vi "Raman Live Tool Set v10.2.2.vi"(1 "Exit":bool, 2 "LiveData":dbl[][](array[numeric]), 3 "RemoteIndicator":bool) -> ()   [LabVIEW 2010]
uses:
  subvi/_TypeDefs/MapFunctions.ctl
  <vilib>/Utility/miscctls.llb/LVPointTypeDef.ctl
  <vilib>/Utility/miscctls.llb/LVStringsAndValuesArrayTypeDef.ctl
  <vilib>/Utility/inputDevices.llb/closeKeyboard.vi
  <vilib>/Utility/inputDevices.llb/keyboardAcquire.vi
  <vilib>/Utility/file.llb/Read From Spreadsheet File (string).vi
  <vilib>/Analysis/NI_AALBase.lvlib
panel:
  in  "MapFunction":T1 caption="Mapping function" items=["Total"=0, "Peak"=4, "Area"=2, "Value"=1, "Ratio"=3]
  in  "CreateMap":bool
  in  "SpectrumCoerce":dbl caption="Limit?"
  out "XY Full Interpol.":cluster{dbl, dbl}[](array[cluster])
  out "Axes":T2
  in  "SpectrumNoise":dbl caption="Noise?"
  in  "SpectrumX":u16(ring) caption="X"
  in  "SpectrumY":u16(ring) caption="Y"
  out "Spectrum":cluster{dbl[], dbl[]}(graph) caption="Current Spectrum"
  in  "MapKeyboard":bool
  in  "MapEditColor":bool caption="Edit Color"
  in  "MapFlipColor":bool caption="Flip Color"
  in  "MapInterpolate":bool
  in  "MapSaveData":bool
  out "Map":dbl[][](graph)
  out "LoadingSpectra":bool
  in  "SourceFile":path caption="Mapping File"
  in  "MapCursorDummy":bool
  out "XY Unique":cluster{"X Unique":dbl[], "Y Unique":dbl[]}
  out "XY Full":cluster{dbl, dbl}[](array[cluster])
  out "Intensities (2D)":dbl[][](array[numeric])
  out "Wavelengths (1D)":dbl[](array[numeric])
  out "MapColorTable":u32[](array[numeric])=[0, 196608, 393216, 589824, 786432, 983040, 1179648, 1376256, 1572864, 1769472, 1966080, 2162688, 2359296, 2555904, 2752512, 2949120, 3145728, 3342336, 3538944, 3735552, 3932160, 4128768, 4325376, 4521984, 4718592, 4915200, 5111808, 5308416, 5505024, 5701632, 5898240, 6094848, 6291456, 6488064, 6684672, 6881280, 7077888, 7274496, 7471104, 7667712, 7864320, 8060928, 8257536, 8454144, 8650752, 8847360, 9043968, 9240576, 9437184, 9633792, 9830400, 10027008, 10223616, 10420224, 10616832, 10813440, 11010048, 11206656, 11403264, 11599872, 11796480, 11993088, 12189696, 12386304, 12582912, 12779520, 12976128, 13172736, 13369344, 13565952, 13762560, 13959168, 14155776, 14352384, 14548992, 14745600, 14942208, 15138816, 15335424, 15532032, 15728640, 15925248, 16121856, 16318464, 16515072, 16711680, 16712448, 16713216, 16713984, 16714752, 16715520, 16716288, 16717056, 16717824, 16718592, 16719360, 16720128, 16720896, 16721664, 16722432, 16723200, 16723968, 16724736, 16725504, 16726272, 16727040, 16727808, 16728576, 16729344, 16730112, 16730880, 16731648, 16732416, 16733184, 16733952, 16734720, 16735488, 16736256, 16737024, 16737792, 16738560, 16739328, 16740096, 16740864, 16741632, 16742400, 16743168, 16743936, 16744704, 16745472, 16746240, 16747008, 16747776, 16748544, 16749312, 16750080, 16750848, 16751616, 16752384, 16753152, 16753920, 16754688, 16755456, 16756224, 16756992, 16757760, 16758528, 16759296, 16760064, 16760832, 16761600, 16762368, 16763136, 16763904, 16764672, 16765440, 16766208, 16766976, 16767744, 16768512, 16769280, 16770048, 16770816, 16771584, 16772352, 16773120, 16773888, 16774656, 16775424, 16776192, 16776960, 16776963, 16776966, 16776969, 16776972, 16776975, 16776977, 16776980, 16776983, 16776986, 16776989, 16776992, 16776995, 16776998, 16777001, 16777004, 16777007, 16777009, 16777012, 16777015, 16777018, 16777021, 16777024, 16777027, 16777030, 16777033, 16777036, 16777038, 16777041, 16777044, 16777047, 16777050, 16777053, 16777056, 16777059, 16777062, 16777065, 16777068, 16777070, 16777073, 16777076, 16777079, 16777082, 16777085, 16777088, 16777091, 16777094, 16777097, 16777100, 16777102, 16777105, 16777108, 16777111, 16777114, 16777117, 16777120, 16777123, 16777126, 16777129, 16777132, 16777134, 16777137, 16777140, 16777143, 16777146, 16777149, 16777152, 16777155, 16777158, 16777161, 16777163, 16777166, 16777169, 16777172, 16777175, 16777178, 16777181, 16777184, 16777187, 16777190, 16777193, 16777195, 16777198, 16777201, 16777204, 16777207]
  out "MapZBounds":cluster{dbl, dbl}
  out "MapData (2D)":dbl[][](array[numeric])
  # "Cursor"
  # "Map Function"
  # "Spectrum"
  # "Raman Live Tool Set"
  # "by A. Schmitz-Wunderlich, P. Candeloro"
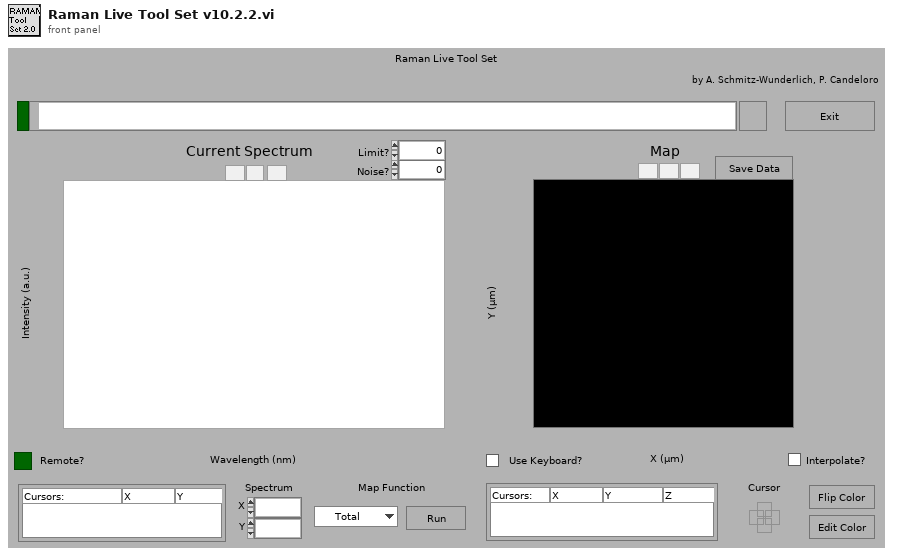
[diagram p1: front panel]
types:
  T1 = typedef "MapFunctions.ctl" = u16
  T2 = cluster{"X":cluster{"Offset":dbl, "Step Size":dbl, "Step Count":i32}, "Y":cluster{"Offset":dbl, "Step Size":dbl, "Step Count":i32}}
  T3 = typedef "LVPointTypeDef.ctl" = cluster{"Horizontal":i16, "Vertical":i16}
  T4 = enum8{"Enabled", "Disabled", "Disabled and Grayed Out"}
  T5 = enum16{"0", "1", "2", "3", "4", "5", "6", "7", "8", "9", "A", "B", "C", "D", "E", "F", "G", "H", "I", "J", "K", "L", "M", "N", "O", "P", "Q", "R", "S", "T", "U", "V", "W", "X", "Y", "Z", "F1", "F2", "F3", "F4", "F5", "F6", "F7", "F8", "F9", "F10", "F11", "F12", "F13", "F14", "F15", "ADD", "BACK", "BACKSLASH", "CAPITAL", "COMMA", "DECIMAL", "DELETE", "DIVIDE", "DOWN", "END", "EQUALS", "ESCAPE", "GRAVE (`)", "HOME", "INSERT", "LBRACKET", "LCONTROL", "LEFT", "L ALT", "LSHIFT", "LWIN", "MINUS", "MULTIPLY", "NEXT", "NUMLOCK", "NUMPAD_0", "NUMPAD_1", "NUMPAD_2", "NUMPAD_3", "NUMPAD_4", "NUMPAD_5", "NUMPAD_6", "NUMPAD_7", "NUMPAD_8", "NUMPAD_9", "PAUSE", "PERIOD", "PRIOR (PG UP)", "RBRACKET", "RCONTROL", "RETURN", "RIGHT", "R ALT", "RSHIFT", "RWIN", "SCROLL", "SEMICOLON", "SLASH", "SPACE", "SUBTRACT", "TAB", "UP", "ENTER (num pad)", "' (quote)"}
  T6 = enum16{"0", "1", "2", "3", "4", "5", "6", "7", "8", "9", "A", "B", "C", "D", "E", "F", "G", "H", "I", "J", "K", "L", "M", "N", "O", "P", "Q", "R", "S", "T", "U", "V", "W", "X", "Y", "Z", "F1", "F2", "F3", "F4", "F5", "F6", "F7", "F8", "F9", "F10", "F11", "F12", "F13", "F14", "F15", "ADD", "BACK", "BACKSLASH", "CAPITAL", "COMMA", "DECIMAL", "DELETE", "DIVIDE", "DOWN", "END", "EQUALS", "ESCAPE", "GRAVE (`)", "HOME", "INSERT", "LBRACKET", "LCONTROL", "LEFT", "L ALT", "LSHIFT", "LWIN", "MINUS", "MULTIPLY", "NEXT", "NUMLOCK", "NUMPAD_0", "NUMPAD_1", "NUMPAD_2", "NUMPAD_3", "NUMPAD_4", "NUMPAD_5", "NUMPAD_6", "NUMPAD_7", "NUMPAD_8", "NUMPAD_9", "PAUSE", "PERIOD", "PRIOR (PG UP)", "RBRACKET", "RCONTROL", "RETURN", "RIGHT", "R ALT", "RSHIFT", "RWIN", "SCROLL", "SEMICOLON", "SLASH", "SPACE", "SUBTRACT", "TAB", "UP", "ENTER (num pad)", "' (quote)"}[]
  T7 = cluster{"Name":string, "Color":u32, "Style":u8, "Point Style":u8, "Name Visible":bool, "Allow Drag":bool, "Cursor Mode":u32, "Plot":i32, "Index":i32, "Position":cluster{"X":dbl, "Y":dbl}, "X Scale":u32, "Y Scale":u32, "Watch Plots":i32[], "Watch All Plots":bool, "Plot Area":i32, "Label Offset":cluster{"X":dbl, "Y":dbl}}
  T8 = cluster{"Name":string, "Color":u32, "Style":u8, "Point Style":u8, "Name Visible":bool, "Allow Drag":bool, "Cursor Mode":u32, "Plot":i32, "Index":i32, "Position":cluster{"X":dbl, "Y":dbl}, "X Scale":u32, "Y Scale":u32, "Watch Plots":i32[], "Watch All Plots":bool, "Plot Area":i32, "Label Offset":cluster{"X":dbl, "Y":dbl}}[]
  T9 = typedef "LVCursorListTypeDef.ctl" = cluster{"Name":string, "Color":u32, "Style":u8, "Point Style":u8, "Name Visible":bool, "Allow Drag":bool, "Cursor Mode":u32, "Plot":i32, "Index":i32, "Position":cluster{"X":dbl, "Y":dbl}, "X Scale":u32, "Y Scale":u32, "Watch Plots":i32[], "Watch All Plots":bool, "Plot Area":i32, "Label Offset":cluster{"X":dbl, "Y":dbl}}[]
  T10 = typedef "LVPointDoubleTypeDef.ctl" = cluster{"Cursor X":dbl, "Cursor Y":dbl}
  T11 = typedef "LVStringsAndValuesArrayTypeDef.ctl" = cluster{"String":string, "Value":ext}[]
  T12 = enum32{"invalid app kind", "Development System", "Run Time System", "Student Edition", "Embedded LabVIEW", "Evaluation", "Custom"}
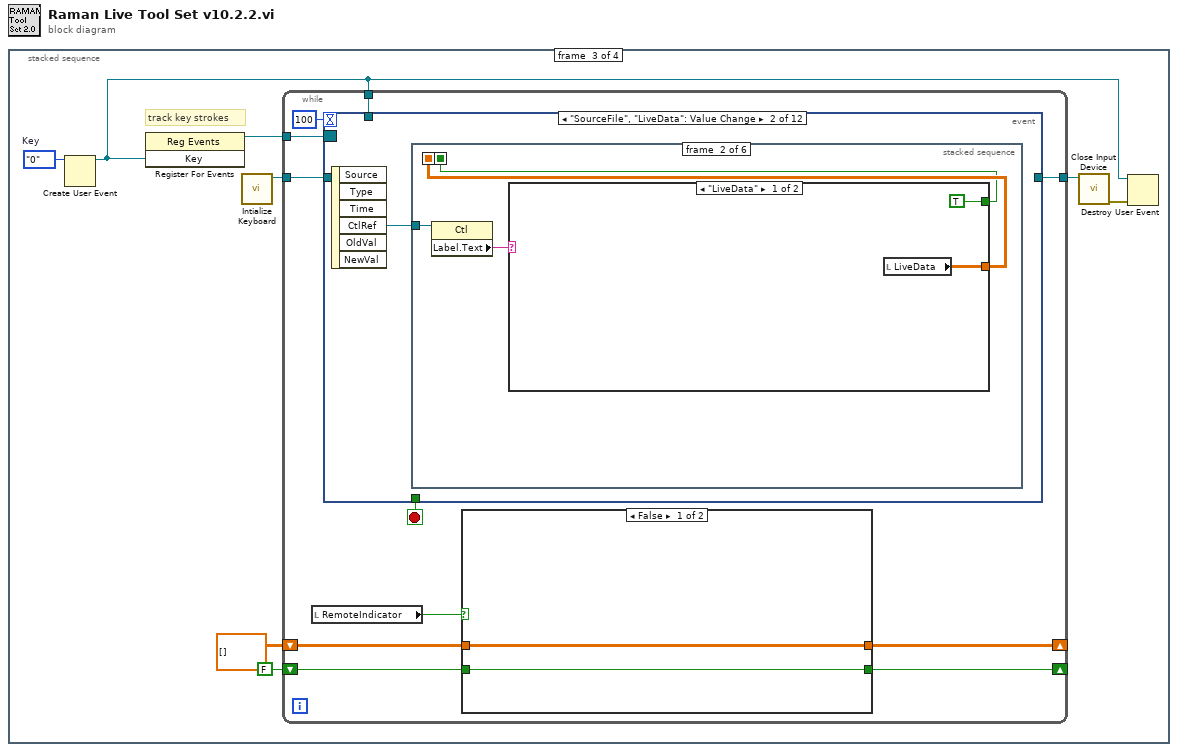
[diagram p0: block diagram]
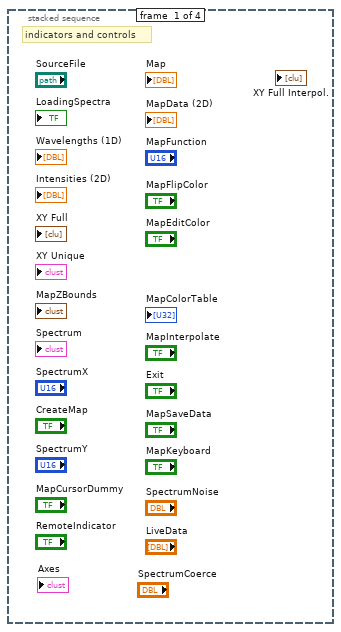
[diagram p2: hidden frame]
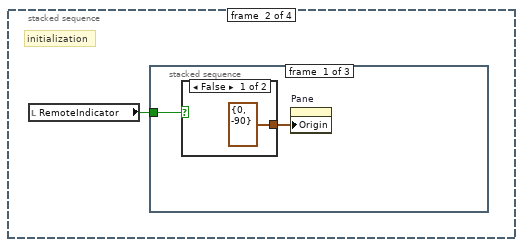
[diagram p3: hidden frame]
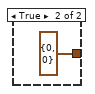
[diagram p4: hidden frame]
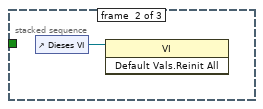
[diagram p5: hidden frame]
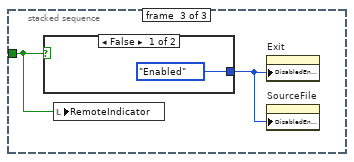
[diagram p6: hidden frame]
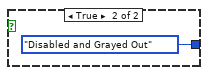
[diagram p7: hidden frame]
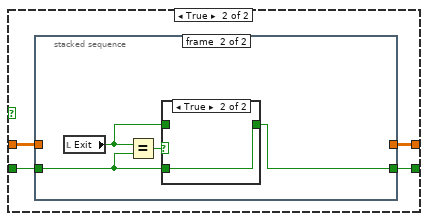
[diagram p8: hidden frame]
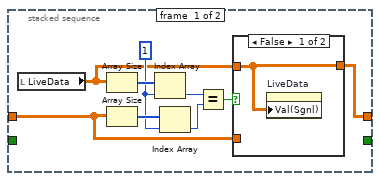
[diagram p9: hidden frame]
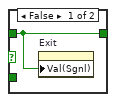
[diagram p11: hidden frame]
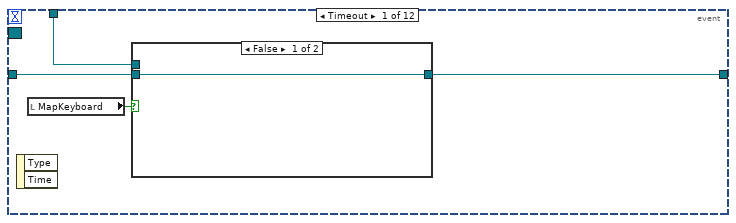
[diagram p12: hidden frame]
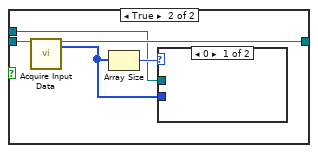
[diagram p13: hidden frame]
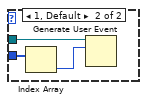
[diagram p14: hidden frame]
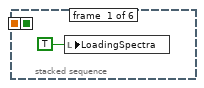
[diagram p15: hidden frame]
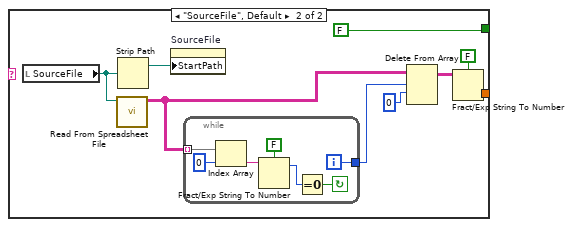
[diagram p16: hidden frame]
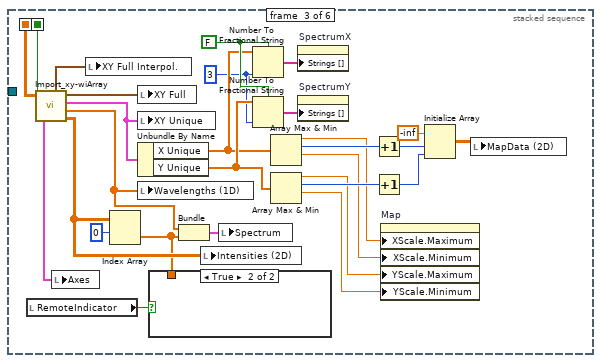
[diagram p17: hidden frame]
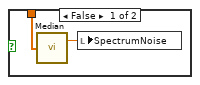
[diagram p18: hidden frame]
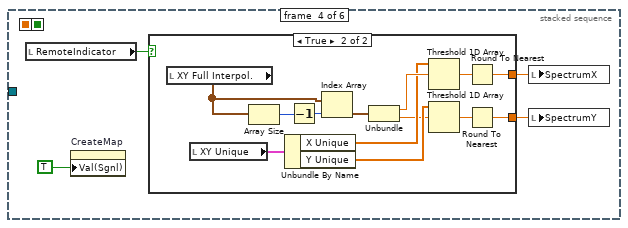
[diagram p19: hidden frame]
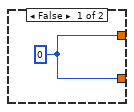
[diagram p20: hidden frame]
diagram:
  n1 = stacked-sequence {
    frame #0 {
      # "indicators and controls"
    }
    frame #1 {
      # "initialization"
      n2 = local read "RemoteIndicator"() -> (w1:bool)
      n3 = stacked-sequence {
        tunnel: w1 -> [w2 _ w7]
        frame #0 {
          n4 = case shown="False" w2 {
            tunnel: [T3 {"Horizontal"=0, "Vertical"=-90} ("Origin") T3 {"Horizontal"=0, "Vertical"=0} ("Origin")] -> w3
            frame False {
            }
            frame True {
            }
          }
          n5 = property on="Pane" class="Pane"("Origin"=w3) -> ()  [unwired: 2 in, 2 out]
        }
        frame #1 {
          n6 = control-ref of="Dieses VI"() -> (w6:refnum<vi>)
          n7 = invoke class="VI" method="Default Vals.Reinit All"(reference=w6) -> ()  [unwired: 2 in, 3 out]
        }
        frame #2 {
          n8 = case shown="False" w7 {
            tunnel: [T4."Enabled" ("Deaktiviert") T4."Disabled and Grayed Out" ("Deaktiviert")] -> w8
            frame False {
            }
            frame True {
            }
          }
          n9 = local write "RemoteIndicator"(w7) -> ()
          n10 = property on="Exit" class="Bool (strict)"("DisabledEnum"=w8) -> ()  [unwired: 2 in, 2 out]
          n11 = property on="SourceFile" class="Path"("DisabledEnum"=w8) -> ()  [unwired: 2 in, 2 out]
        }
      }
    }
    frame #2 {
      w18 = T5."0"  # Key
      # "track key strokes"
      n12 = Create User Event(user event datatype=w18) -> (user event=w15:refnum<user-event>)  [unwired: 1 in, 1 out]
      n13 = register-events(w15) -> (reference out=w16:refnum<event-registration>)  [unwired: 2 in, 1 out]
      n14 = call <vilib>:"Intialize Keyboard.vi"() -> ("device ID"=w14:refnum<k1>)  [unwired: 10 in, 1 out]
      n15 = while {
        tunnel: w16 -> [w28]
        tunnel: w15 -> [w27]
        tunnel: w14 -> [w26]
        tunnel: [w25] -> w13
        shift-right: [w21] -> _
        shift-left: dbl[][] [] ("LiveData") -> [w22]
        shift-right: [w19] -> _
        shift-left: FALSE -> [w20]
        stop <- w29 stop-if-true
        n16 = local read "RemoteIndicator"() -> (w23:bool)
        n17 = event shown="[1] \"SourceFile\", \"LiveData\": Value Change" {
          selector: w28 -> [_ _ _ _ _ _ _ _ _ _ _ _]
          dyn-events: _ -> [_ _ _ _ _ _ _ _ _ _ _ _]
          timeout: 100 -> [_ _ _ _ _ _ _ _ _ _ _ _]
          tunnel: [_ _ _ _ _ _ _ _ _ _ _ w341] -> w29
          tunnel: w27 -> [w56 _ _ _ _ _ _ _ _ _ _ _]
          tunnel: w26 -> [w55 _ _ _ _ _ _ _ _ _ _ _]
          tunnel: [w53 _ _ _ _ _ _ _ _ _ _ _] -> w25
          event Timeout {
            n18 = event-data() -> ()  [unwired: 1 in, 2 out]
            n19 = local read "MapKeyboard"() -> (w54:bool)
            n20 = case shown="False" w54 {
              tunnel: [w57 w62] -> w53
              tunnel: w56 -> [_ w59]
              tunnel: w55 -> [w57 w58]
              frame False {
              }
              frame True {
                n21 = call-poly <vilib>:"Acquire Input Data.vi"("device ID"=w58) -> ("device ID"=w62:refnum<k1>, "keys pressed"=w61:T6)  [unwired: 16 in, 1 out]
                n22 = Array Size(array=w61) -> (size(s)=w60:i32)
                n23 = case shown="0" w60 {
                  tunnel: w59 -> [_ w65]
                  tunnel: w61 -> [_ w63]
                  frame 0 {
                  }
                  frame 1, Default {
                    n24 = Index Array(array=w63) -> (element=w64:T5)  [unwired: 1 in]
                    n25 = Generate User Event(user event=w65, event data cluster=w64) -> ()  [unwired: 1 in, 2 out]
                  }
                }
              }
            }
          }
          event "SourceFile", "LiveData": Value Change {
            n26 = event-data() -> ("CtlRef"=w66:refnum<vi>)  [unwired: 1 in, 5 out]
            n27 = stacked-sequence {
              seq-local: [_ w69 _ _ _ _] -> [_ _ w99 _ _ _]
              seq-local: [_ w68 _ _ _ _] -> [_ _ w92 _ _ _]
              tunnel: w66 -> [_ w71 _ _ _ _]
              frame #0 {
                n28 = local write "LoadingSpectra"(TRUE ("Loading\nSpectra")) -> ()
              }
              frame #1 {
                n29 = property class="Ctl"(reference=w71) -> ("Label.Text"=w70:string)  [unwired: 1 in, 2 out]
                n30 = case shown="\"LiveData\"" w70 {
                  tunnel: [w73 w78] -> w69
                  tunnel: [TRUE FALSE] -> w68
                  frame "LiveData" {
                    n31 = local read "LiveData"() -> (w73:dbl[][])
                  }
                  frame "SourceFile", Default {
                    n32 = local read "SourceFile"() -> (w80:path)
                    n33 = call-poly <vilib>:"Read From Spreadsheet File.vi"("file path (dialog if empty)"=w80) -> ("all rows"=w76:string[][])  [unwired: 6 in, 4 out]
                    n34 = Strip Path(path=w80) -> (stripped path=w82:path)  [unwired: 1 out]
                    n35 = property on="SourceFile" class="Path"("StartPath"=w82) -> ()  [unwired: 2 in, 2 out]
                    n36 = while {
                      tunnel: w76 -> [w89] mode=indexing
                      tunnel: [w83] -> w75
                      i -> [w83]
                      stop <- w84 continue-if-true
                      n37 = Index Array(array=w89, index=0) -> (element=w86:string)
                      n38 = Fract/Exp String To Number(use system decimal point (T)=FALSE, string=w86) -> (offset past number=w85:i32)  [unwired: 2 in, 1 out]
                      n39 = Equal To 0?(x=w85) -> (x = 0?=w84:bool)
                    }
                    n40 = Delete From Array(array=w76, length=w75, index (row)=0) -> (array with subset deleted=w77:string[][])  [unwired: 1 in, 1 out]
                    n41 = Fract/Exp String To Number(use system decimal point (T)=FALSE, string=w77) -> (number=w78:dbl[][])  [unwired: 2 in, 1 out]
                  }
                }
              }
              frame #2 {
                w106 = i16 3 ("Genauigkeit (6)")
                w113 = FALSE ("Systemdezimalzeichen verwenden (T)")
                n42 = local read "RemoteIndicator"() -> (w93:bool)
                n43 = call "Import_xy-wiArray.vi"("InputArray"=w99, "Uniform"=w92) -> ("XY Full"=w91:cluster{dbl, dbl}[], "XY Unique"=w96:cluster{"X Unique":dbl[], "Y Unique":dbl[]}, "Wavelength"=w97:dbl[], "Intensity"=w98:dbl[][], "XY Full Interpol."=w90:cluster{dbl, dbl}[], "Axes"=w94:T2)
                n44 = local write "Axes"(w94) -> ()
                n45 = local write "XY Full Interpol."(w90) -> ()
                n46 = Index Array(array=w98, index (row)=0 ("Index (Zeile)")) -> (element=w95:dbl[])  [unwired: 1 in]
                n47 = local write "XY Full"(w91) -> ()
                n48 = local write "XY Unique"(w96) -> ()
                n49 = Unbundle By Name(w96) -> ("X Unique"=w107:dbl[], "Y Unique"=w108:dbl[])
                n50 = local write "Wavelengths (1D)"(w97) -> ()
                n51 = case shown="True" w93 {
                  tunnel: w95 -> [w118 _]
                  frame False {
                    n52 = call <vilib>:"Median.vi"("X"=w118) -> ("median"=w119:dbl)  [unwired: 1 out]
                    n53 = local write "SpectrumNoise"(w119) -> ()
                  }
                  frame True {
                  }
                }
                n54 = Bundle("Wavelength"=w97, "Intensity"=w95) -> (w117:cluster{"Wavelength":dbl[], "Intensity":dbl[]})  [unwired: 1 in]
                n55 = local write "Intensities (2D)"(w98) -> ()
                n56 = local write "Spectrum"(w117) -> ()
                n57 = Number To Fractional String(use system decimal point (T)=w113, number=w107, precision (6)=w106) -> (F-format string=w110:string[])  [unwired: 1 in]
                n58 = Number To Fractional String(use system decimal point (T)=w113, number=w108, precision (6)=w106) -> (F-format string=w109:string[])  [unwired: 1 in]
                n59 = Array Max & Min(array=w107) -> (max value=w103:dbl, max index (indices)=w105:i32, min value=w102:dbl)  [unwired: 1 out]
                n60 = Array Max & Min(array=w108) -> (max value=w101:dbl, max index (indices)=w104:i32, min value=w100:dbl)  [unwired: 1 out]
                n61 = property on="SpectrumX" class="Ring (strict)"("Strings []"=w110) -> ()  [unwired: 2 in, 2 out]
                n62 = property on="SpectrumY" class="Ring (strict)"("Strings []"=w109) -> ()  [unwired: 2 in, 2 out]
                n63 = Increment(x=w105) -> (x+1=w114:i32)
                n64 = Increment(x=w104) -> (x+1=w115:i32)
                n65 = property on="Map" class="IntGraph (strict)"("XScale.Maximum"=w103, "XScale.Minimum"=w102, "YScale.Maximum"=w101, "YScale.Minimum"=w100) -> ()  [unwired: 2 in, 2 out]
                n66 = Initialize Array(-inf, w114, w115) -> (w112:dbl[][])
                n67 = local write "MapData (2D)"(w112) -> ()
              }
              frame #3 {
                n68 = local read "RemoteIndicator"() -> (w123:bool)
                n69 = property on="CreateMap" class="Bool (strict)"("Val(Sgnl)"=TRUE ("Wert (signalisierend)")) -> ()  [unwired: 2 in, 2 out]
                n70 = case shown="True" w123 {
                  tunnel: [w124 w125] -> w122
                  tunnel: [w124 w126] -> w121
                  frame False {
                    w124 = 0
                  }
                  frame True {
                    n71 = local read "XY Full Interpol."() -> (w134:cluster{dbl, dbl}[])
                    n72 = local read "XY Unique"() -> (w137:cluster{"X Unique":dbl[], "Y Unique":dbl[]})
                    n73 = Array Size(array=w134) -> (size(s)=w136:i32)
                    n74 = Unbundle By Name(w137) -> ("X Unique"=w130:dbl[], "Y Unique"=w129:dbl[])
                    n75 = Decrement(x=w136) -> (x-1=w135:i32)
                    n76 = Index Array(array=w134, index=w135) -> (element=w133:cluster{dbl, dbl})
                    n77 = Unbundle(w133) -> (w131:dbl, w128:dbl)
                    n78 = Threshold 1D Array(2:w131, 3:w130) -> (0:w132:dbl)  [unwired: 1 in]
                    n79 = Threshold 1D Array(2:w128, 3:w129) -> (0:w127:dbl)  [unwired: 1 in]
                    n80 = Round To Nearest(number=w132) -> (nearest integer value=w125:dbl)
                    n81 = Round To Nearest(number=w127) -> (nearest integer value=w126:dbl)
                  }
                }
                n82 = local write "SpectrumX"(w122) -> ()
                n83 = local write "SpectrumY"(w121) -> ()
              }
              frame #4 {
                w147 = i8 2 ("y")
                w155 = T7 {"Name"="cursor", "Color"=1985280, "Style"=2, "Point Style"=6, "Name Visible"=FALSE, "Allow Drag"=TRUE, "Cursor Mode"=0, "Plot"=0, "Index"=0, "Position"={"X"=0.0, "Y"=0.0}, "X Scale"=0, "Y Scale"=0, "Watch Plots"=[], "Watch All Plots"=FALSE, "Plot Area"=0, "Label Offset"={"X"=0.0, "Y"=0.0}}  # cursorConst
                n84 = local read "Axes"() -> (w151:T2)
                n85 = Unbundle By Name(w151) -> ("X.Offset"=w150:dbl, "X.Step Size"=w149:dbl, "Y.Offset"=w146:dbl, "Y.Step Size"=w148:dbl)
                n86 = Divide(x=w149, y=w147) -> (x/y=w145:dbl)
                n87 = Divide(x=w148, y=w147) -> (x/y=w144:dbl)
                n88 = Add(x=w150, y=w145) -> (x+y=w142:dbl)
                n89 = Add(x=w146, y=w144) -> (x+y=w143:dbl)
                n90 = Bundle(w142, w143) -> (w140:cluster{dbl, dbl})  [unwired: 1 in]
                n91 = Bundle By Name(cluster=w155, "Name"="Spot", "Cursor Mode"=u32 0, "Position"=w140) -> (w139:T7)
                n92 = Build Array(w139) -> (w138:T8)
                n93 = property on="Map" class="IntGraph (strict)"("CrsrLis"=w138, "Cursor.Cursor Style"=u8 8, "Cursor.Cursor Point Style"=u8 5, "Cursor.Cursor Color"=u32 16448250 ("Color")) -> ()  [unwired: 2 in, 2 out]
              }
              frame #5 {
                n94 = local write "LoadingSpectra"(FALSE ("Loading\nSpectra")) -> ()
              }
            }
          }
          event "CreateMap": Value Change {
            n95 = event-data() -> ("NewVal"=w158:bool)  [unwired: 1 in, 5 out]
            n96 = case shown="True" w158 {
              frame False {
              }
              frame True {
                n97 = stacked-sequence {
                  frame #0 {
                    n98 = local read "SpectrumCoerce"() -> (w163:dbl)
                    n99 = local read "SpectrumNoise"() -> (w166:dbl)
                    n100 = local read "Intensities (2D)"() -> (w159:dbl[][])
                    n101 = property on="Spectrum" class="XYGraph (strict)"() -> ("CrsrList"=w170:T9)  [unwired: 2 in, 2 out]
                    n102 = Equal To 0?(x=w163) -> (x = 0?=w162:bool)
                    n103 = Subtract(x=w159, y=w166) -> (x-y=w160:dbl[][])
                    n104 = local read "XY Full Interpol."() -> (w165:cluster{dbl, dbl}[])
                    n105 = case shown="False" w162 {
                      tunnel: w163 -> [w181 _]
                      tunnel: [w180 w182] -> w161
                      tunnel: w160 -> [w179 w182]
                      frame False {
                        n106 = In Range and Coerce(upper limit=w181, x=w179, lower limit=-1000.0 ("SpectrumCoerce")) -> (coerced(x)=w180:dbl[][])  [unwired: 1 out]
                      }
                      frame True {
                      }
                    }
                    n107 = local read "Wavelengths (1D)"() -> (w177:dbl[])
                    n108 = local read "MapFunction"() -> (w167:T1)
                    n109 = Index Array(array=w170, index=0 ("Index")) -> (element=w173:T7)
                    n110 = Index Array(array=w170, index=1 ("Index")) -> (element=w174:T7)
                    n111 = Unbundle By Name(w173) -> ("Position.X"=w169:dbl)
                    n112 = Unbundle By Name(w174) -> ("Position.X"=w168:dbl)
                    n113 = local read "XY Unique"() -> (w164:cluster{"X Unique":dbl[], "Y Unique":dbl[]})
                    n114 = call "Map_spectra2MapData.vi"("Intensity"=w161, "Wavelength"=w177, "XY Unique"=w164, "XY Full"=w165, "MapFunction"=w167, "X1"=w169, "X2"=w168) -> ("MapZBounds"=w175:cluster{sgl, sgl}, "MapData"=w176:sgl[][])  [unwired: 2 in]
                    n115 = local write "MapData (2D)"(w176) -> ()
                    n116 = local write "MapZBounds"(w175) -> ()
                    n117 = property on="Map" class="IntGraph (strict)"("Val(Sgnl)"=w176) -> ()  [unwired: 2 in, 2 out]
                  }
                  frame #1 {
                    n118 = local read "SpectrumX"() -> (w184:u16)
                    n119 = local write "CreateMap"(FALSE ("Value")) -> ()
                    n120 = property on="SpectrumX" class="Ring (strict)"("Val(Sgnl)"=w184) -> ()  [unwired: 2 in, 2 out]
                  }
                }
              }
            }
          }
          event "Map", "MapInterpolate", "MapFlipColor": Value Change {
            n121 = event-data() -> ()  [unwired: 1 in, 6 out]
            n122 = stacked-sequence {
              seq-local: [w185 _ _ _ _] -> [_ _ w210 _ _]
              frame #0 {
                n123 = local read "MapInterpolate"() -> (w190:bool)
                n124 = local read "MapData (2D)"() -> (w189:dbl[][])
                n125 = local read "XY Unique"() -> (w186:cluster{"X Unique":dbl[], "Y Unique":dbl[]})
                n126 = local read "Axes"() -> (w188:T2)
                n127 = case shown="True" w190 {
                  tunnel: [w192 w196] -> w187
                  tunnel: w189 -> [w192 w197]
                  tunnel: w188 -> [w191 _]
                  tunnel: w186 -> [_ w194]
                  tunnel: [w191 w193] -> w185
                  frame False {
                  }
                  frame True {
                    n128 = call "Map_interpolateXYZ.vi"("Level"=3, "MapData (2D)"=w197, "XY Unique"=w194) -> ("Z Interpoliert"=w196:dbl[][], "Axes"=w193:T2)  [unwired: 1 out]
                  }
                }
                n129 = local write "Map"(w187) -> ()
              }
              frame #1 {
                w205 = u32 0 ("Color")
                n130 = local read "MapColorTable"() -> (w203:u32[])
                n131 = local read "MapZBounds"() -> (w204:cluster{dbl, dbl})
                n132 = local read "MapFlipColor"() -> (w202:bool)
                n133 = Unbundle(w204) -> (w208:dbl, w201:dbl)
                n134 = Greater Than 0?(x=w201) -> (x > 0?=w199:bool)
                n135 = Reverse 1D Array(array=w203) -> (reversed array=w207:u32[])
                n136 = Select(t=w201, s=w199, f=0.0) -> (s? t:f=w198:dbl)
                n137 = Select(t=w207, s=w202, f=w203) -> (s? t:f=w206:u32[])
                n138 = property on="Map" class="IntGraph (strict)"("ZScale.Interpolate Color"=TRUE ("Z Scale.Interpolate Color"), "ZScale.Maximum"=w208, "ZScale.Minimum"=w198, "Color Table"=w206, "ZScale.High Color"=w205, "ZScale.Low Color"=w205) -> ()  [unwired: 2 in, 2 out]
              }
              frame #2 {
                n139 = Unbundle By Name(w210) -> ("X.Offset"=w214:dbl, "X.Step Size"=w213:dbl, "Y.Offset"=w212:dbl, "Y.Step Size"=w211:dbl)
                n140 = property on="Map" class="IntGraph (strict)"("XScale.Offset"=w214, "XScale.Multiplier"=w213, "YScale.Offset"=w212, "YScale.Multiplier"=w211) -> ()  [unwired: 2 in, 2 out]
              }
              frame #3 {
                w215 = u8 1 ("X-Achse.Achsenanpassung")
                n141 = property on="Map" class="IntGraph (strict)"("XScale.ScaleFit"=w215, "YScale.ScaleFit"=w215, "ZScale.ScaleFit"=u8 0 ("Z-Achse.Achsenanpassung")) -> ()  [unwired: 2 in, 2 out]
              }
              frame #4 {
                n142 = local read "SpectrumX"() -> (w217:u16)
                n143 = property on="SpectrumX" class="Ring (strict)"("Val(Sgnl)"=w217) -> ()  [unwired: 2 in, 2 out]
              }
            }
          }
          event "MapEditColor": Value Change {
            n144 = event-data() -> ("NewVal"=w218:bool)  [unwired: 1 in, 5 out]
            n145 = case shown="True" w218 {
              frame False {
              }
              frame True {
                n146 = flat-sequence {
                  frame #0 {
                    n147 = local read "MapColorTable"() -> (w219:u32[])
                    n148 = call "MapColor_makeRamp.vi"("ColorMap\narray IN"=w219) -> ("ColorMap\narray OUT"=w220:u32[])
                    n149 = local write "MapColorTable"(w220) -> ()
                  }
                  frame #1 {
                    n150 = local read "MapData (2D)"() -> (w222:dbl[][])
                    n151 = local write "MapEditColor"(FALSE ("Value")) -> ()
                    n152 = property on="Map" class="IntGraph (strict)"("Val(Sgnl)"=w222) -> ()  [unwired: 2 in, 2 out]
                  }
                }
              }
            }
          }
          event "MapSaveData": Value Change {
            n153 = event-data() -> ("NewVal"=w223:bool)  [unwired: 1 in, 5 out]
            n154 = case shown="True" w223 {
              frame False {
              }
              frame True {
                n155 = flat-sequence {
                  frame #0 {
                    n156 = property on="MapFunction" class="Ring (strict)"() -> ("RingText.Text"=w225:string)  [unwired: 2 in, 2 out]
                    n157 = local read "SourceFile"() -> (w224:path)
                    n158 = control-ref of="Spectrum"() -> (w226:refnum<vi>)
                    n159 = call "Export_mapFileName.vi"("MapFunctionStr"=w225, "Spectrum"=w226, "SourceFile"=w224) -> ("Dateipfad"=w227:path)
                    n160 = local read "XY Full Interpol."() -> (w228:cluster{dbl, dbl}[])
                    n161 = local read "Map"() -> (w229:dbl[][])
                    n162 = call "Export_map2Text v10.2.vi"("MapData (2D)"=w229, "XY Full Interpolated"=w228, "ExportPath"=w227) -> ()  [unwired: 1 in]
                  }
                  frame #1 {
                    n163 = local write "MapSaveData"(FALSE ("Value")) -> ()
                    n164 = Wait (ms)(milliseconds to wait=u32 300) -> ()  [unwired: 1 out]
                  }
                }
              }
            }
          }
          event Value Change {
            n165 = event-data() -> ()  [unwired: 1 in, 6 out]
            n166 = local read "MapFunction"() -> (w232:T1)
            n167 = control-ref of="Spectrum"() -> (w233:refnum<vi>)
            n168 = call "SpectrumCursor_init.vi"("MapFunction"=w232, "Spectrum"=w233) -> ()  [unwired: 1 in]
          }
          event "SpectrumY", "SpectrumX", "SpectrumNoise", "SpectrumCoerce": Value Change {
            n169 = event-data() -> ()  [unwired: 1 in, 6 out]
            n170 = local read "XY Unique"() -> (w251:cluster{"X Unique":dbl[], "Y Unique":dbl[]})
            n171 = local read "SpectrumX"() -> (w246:u16)
            n172 = local read "SpectrumY"() -> (w247:u16)
            n173 = Unbundle By Name(w251) -> ("X Unique"=w249:dbl[], "Y Unique"=w248:dbl[])
            n174 = local read "Intensities (2D)"() -> (w253:dbl[][])
            n175 = local read "SpectrumCoerce"() -> (w237:dbl)
            n176 = local read "XY Full Interpol."() -> (w239:cluster{dbl, dbl}[])
            n177 = local read "SpectrumNoise"() -> (w250:dbl)
            n178 = Index Array(array=w249, index=w246) -> (element=w256:dbl)
            n179 = Index Array(array=w248, index=w247) -> (element=w255:dbl)
            n180 = Bundle(cluster=cluster{dbl, dbl} {0.0, 0.0} ("Element"), w256, w255) -> (w242:cluster{dbl, dbl})
            n181 = Equal To 0?(x=w237) -> (x = 0?=w238:bool)
            n182 = property on="Map" class="IntGraph (strict)"("Cursor.Cursor Position"=w242) -> ()  [unwired: 2 in, 2 out]
            n183 = while {
              tunnel: w239 -> [w268] mode=indexing
              tunnel: w242 -> [w269]
              tunnel: [w267] -> w244
              tunnel: [w264] -> w241
              tunnel: w239 -> [w265]
              i -> [w267]
              stop <- w262 stop-if-true
              n184 = Array Size(array=w265) -> (size(s)=w266:i32)
              n185 = Equal?(x=w268, y=w269) -> (x = y?=w264:bool)
              n186 = Greater?(x=w267, y=w266) -> (0:w263:bool)
              n187 = Or(x=w263, y=w264) -> (x .or. y?=w262:bool)
            }
            n188 = local read "Wavelengths (1D)"() -> (w254:dbl[])
            n189 = Select(t=w244, s=w241, f=u8 0) -> (s? t:f=w240:i32)
            n190 = Index Array(array=w253, index (row)=w240) -> (element=w236:dbl[])  [unwired: 1 in]
            n191 = Subtract(x=w236, y=w250) -> (x-y=w235:dbl[])
            n192 = case shown="False" w238 {
              tunnel: w237 -> [w260 _]
              tunnel: w235 -> [w259 w261]
              tunnel: [w258 w261] -> w234
              frame False {
                n193 = In Range and Coerce(upper limit=w260, x=w259, lower limit=-1000.0 ("SpectrumCoerce")) -> (coerced(x)=w258:dbl[])  [unwired: 1 out]
              }
              frame True {
              }
            }
            n194 = Bundle("Wavelengths (1D)"=w254, w234) -> (w252:cluster{"Wavelengths (1D)":dbl[], dbl[]})  [unwired: 1 in]
            n195 = local write "Spectrum"(w252) -> ()
          }
          event "Map": Cursor Release; "MapCursorDummy": Value Change {
            n196 = event-data() -> ()  [unwired: 1 in, 4 out]
            n197 = property on="Map" class="IntGraph (strict)" props=["Cursor", "Cursor Position", "Cursor", "Cursor Position"]() -> ("Cursor.Cursor Position"=w279:T10)  [unwired: 2 in, 3 out]
            n198 = local read "XY Unique"() -> (w284:cluster{"X Unique":dbl[], "Y Unique":dbl[]})
            n199 = Unbundle By Name(w284) -> ("X Unique"=w272:dbl[], "Y Unique"=w273:dbl[])
            n200 = Unbundle By Name(w279) -> ("Cursor X"=w283:dbl, "Cursor Y"=w282:dbl)
            n201 = Threshold 1D Array(2:w283, 3:w272) -> (0:w278:dbl)  [unwired: 1 in]
            n202 = Threshold 1D Array(2:w282, 3:w273) -> (0:w277:dbl)  [unwired: 1 in]
            n203 = Round To Nearest(number=w278) -> (nearest integer value=w280:dbl)
            n204 = Round To Nearest(number=w277) -> (nearest integer value=w281:dbl)
            n205 = To Unsigned Word Integer(number=w280) -> (unsigned 16bit integer=w270:u16)
            n206 = To Unsigned Word Integer(number=w281) -> (unsigned 16bit integer=w271:u16)
            n207 = Not Equal?(x=w270, y=w278) -> (x != y?=w275:bool)
            n208 = Not Equal?(x=w271, y=w277) -> (x != y?=w276:bool)
            n209 = property on="SpectrumX" class="Ring (strict)"("Val(Sgnl)"=w270) -> ()  [unwired: 2 in, 2 out]
            n210 = property on="SpectrumY" class="Ring (strict)"("Val(Sgnl)"=w271) -> ()  [unwired: 2 in, 2 out]
            n211 = Or(x=w275, y=w276) -> (x .or. y?=w274:bool)
            n212 = case shown="True" w274 {
              tunnel: w273 -> [_ w288]
              tunnel: w272 -> [_ w287]
              tunnel: w271 -> [_ w286]
              tunnel: w270 -> [_ w285]
              frame False {
              }
              frame True {
                n213 = Index Array(array=w287, index=w285) -> (element=w290:dbl)
                n214 = Index Array(array=w288, index=w286) -> (element=w291:dbl)
                n215 = Bundle(w290, w291) -> (w289:cluster{dbl, dbl})  [unwired: 1 in]
                n216 = property on="Map" class="IntGraph (strict)"("Cursor.Cursor Position"=w289) -> ()  [unwired: 2 in, 2 out]
              }
            }
          }
          event "Spectrum": Cursor Release {
            n217 = event-data() -> ()  [unwired: 1 in, 9 out]
            n218 = local read "MapFunction"() -> (w292:T1)
            n219 = control-ref of="Spectrum"() -> (w293:refnum<vi>)
            n220 = call "SpectrumCursor_set.vi"("MapFunction"=w292, "Spectrum"=w293) -> ()
          }
          event User Event {
            n221 = event-data() -> ("Key"=w300:T5)  [unwired: 1 in, 4 out]
            n222 = property on="Map" class="IntGraph (strict)"() -> ("Cursor.Cursor Position"=w301:T10)  [unwired: 2 in, 2 out]
            n223 = local read "Axes"() -> (w294:T2)
            n224 = property on="Map" class="IntGraph (strict)"() -> ("XScale.Maximum"=w305:dbl, "YScale.Maximum"=w304:dbl, "XScale.Minimum"=w303:dbl, "YScale.Minimum"=w302:dbl)  [unwired: 2 in, 2 out]
            n225 = Unbundle By Name(w294) -> ("X.Step Size"=w298:dbl, "Y.Step Size"=w297:dbl)
            n226 = Unbundle By Name(w301) -> ("Cursor X"=w306:dbl, "Cursor Y"=w307:dbl)
            n227 = case shown="\"DOWN\"" w300 {
              tunnel: w303 -> [_ w313 _ _ _]
              tunnel: w305 -> [_ _ w320 _ _]
              tunnel: w304 -> [_ _ _ w327 _]
              tunnel: w302 -> [_ _ _ _ w334]
              tunnel: w306 -> [w311 w312 w319 w331 w338]
              tunnel: w307 -> [w310 w317 w324 w326 w333]
              tunnel: [w310 w317 w324 w330 w337] -> w308
              tunnel: [w311 w316 w323 w331 w338] -> w309
              tunnel: w298 -> [_ w315 w322 _ _]
              tunnel: w297 -> [_ _ _ w328 w335]
              frame "0", Default {
              }
              frame "LEFT" {
                n228 = Subtract(x=w312, y=w315) -> (x-y=w314:dbl)
                n229 = Greater Or Equal?(x=w313, y=w314) -> (x >= y?=w318:bool)
                n230 = Select(t=w312, s=w318, f=w314) -> (s? t:f=w316:dbl)
              }
              frame "RIGHT" {
                n231 = Add(x=w319, y=w322) -> (x+y=w321:dbl)
                n232 = Greater Or Equal?(x=w320, y=w321) -> (x >= y?=w325:bool)
                n233 = Select(t=w321, s=w325, f=w319) -> (s? t:f=w323:dbl)
              }
              frame "UP" {
                n234 = Add(x=w326, y=w328) -> (x+y=w329:dbl)
                n235 = Less Or Equal?(x=w327, y=w329) -> (x <= y?=w332:bool)
                n236 = Select(t=w326, s=w332, f=w329) -> (s? t:f=w330:dbl)
              }
              frame "DOWN" {
                n237 = Subtract(x=w333, y=w335) -> (x-y=w336:dbl)
                n238 = Greater Or Equal?(x=w334, y=w336) -> (x >= y?=w339:bool)
                n239 = Select(t=w333, s=w339, f=w336) -> (s? t:f=w337:dbl)
              }
            }
            n240 = Bundle("Cursor X"=w309, "Cursor Y"=w308) -> (w299:cluster{"Cursor X":dbl, "Cursor Y":dbl})  [unwired: 1 in]
            n241 = local read "MapCursorDummy"() -> (w295:bool)
            n242 = property on="Map" class="IntGraph (strict)"("Cursor.Cursor Position"=w299) -> (error out=w296:errorcluster)  [unwired: 2 in, 1 out]
            n243 = property on="MapCursorDummy" class="Bool (strict)"(error in=w296, "Val(Sgnl)"=w295) -> ()  [unwired: 1 in, 2 out]
          }
          event "Exit": Value Change {
            n244 = event-data() -> ("OldVal"=w340:bool, "NewVal"=w341:bool)  [unwired: 1 in, 4 out]
            n245 = local write "Exit"(w340) -> ()
          }
        }
        n246 = case shown="False" w23 {
          tunnel: w22 -> [w31 w35]
          tunnel: [w31 w34] -> w21
          tunnel: w20 -> [w30 w33]
          tunnel: [w30 w32] -> w19
          frame False {
          }
          frame True {
            n247 = stacked-sequence {
              tunnel: w35 -> [w39 _]
              tunnel: [w38 _] -> w34
              tunnel: w33 -> [_ w47]
              tunnel: [_ w49] -> w32
              frame #0 {
                w42 = 1 ("Index")
                n248 = local read "LiveData"() -> (w40:dbl[][])
                n249 = Array Size(array=w40) -> (size(s)=w43:i32[])
                n250 = Array Size(array=w39) -> (size(s)=w44:i32[])
                n251 = Index Array(array=w43, index=w42) -> (element=w37:i32)
                n252 = Index Array(array=w44, index=w42) -> (element=w36:i32)
                n253 = Equal?(x=w37, y=w36) -> (x = y?=w41:bool)
                n254 = case shown="False" w41 {
                  tunnel: [w45 w46] -> w38
                  tunnel: w39 -> [_ w46]
                  tunnel: w40 -> [w45 _]
                  frame False {
                    n255 = property on="LiveData" class="Arr (strict)"("Val(Sgnl)"=w45) -> ()  [unwired: 2 in, 2 out]
                  }
                  frame True {
                  }
                }
              }
              frame #1 {
                n256 = local read "Exit"() -> (w48:bool)
                n257 = Equal?(x=w48, y=w47) -> (x = y?=w50:bool)
                n258 = case shown="True" w50 {
                  tunnel: [w51 w52] -> w49
                  tunnel: w47 -> [_ w52]
                  tunnel: w48 -> [w51 _]
                  frame False {
                    n259 = property on="Exit" class="Bool (strict)"("Val(Sgnl)"=w51) -> ()  [unwired: 2 in, 2 out]
                  }
                  frame True {
                  }
                }
              }
            }
          }
        }
      }
      n260 = call-poly <vilib>:"Close Input Device.vi"("device ID"=w13) -> ("error out"=w17:errorcluster)  [unwired: 9 in]
      n261 = Destroy User Event(user event=w15, error in=w17) -> ()  [unwired: 1 out]
    }
    frame #3 {
      w344 = T4."Enabled" ("Deaktiviert")
      w345 = T11 [] ("Strings und Werte []")
      w346 = T8 [] ("Cursor List")
      # "reset and shutdown"
      n262 = control-ref of="Dieses VI"() -> (w347:refnum<vi>)
      n263 = invoke class="VI" method="Default Vals.Reinit All"(reference=w347) -> (reference out=w342:refnum<vi>)  [unwired: 2 in, 2 out]
      n264 = property on="SpectrumY" class="Ring (strict)"("StringsAndValues[]"=w345) -> ()  [unwired: 2 in, 2 out]
      n265 = property on="SpectrumX" class="Ring (strict)"("StringsAndValues[]"=w345) -> ()  [unwired: 2 in, 2 out]
      n266 = property on="SourceFile" class="Path"("DisabledEnum"=w344) -> ()  [unwired: 2 in, 2 out]
      n267 = property on="Exit" class="Bool (strict)"("DisabledEnum"=w344) -> ()  [unwired: 2 in, 2 out]
      n268 = property on="Map" class="IntGraph (strict)"("CrsrLis"=w346) -> ()  [unwired: 2 in, 2 out]
      n269 = property on="Spectrum" class="XYGraph (strict)"("CrsrList"=w346) -> ()  [unwired: 2 in, 2 out]
      n270 = property class="App"() -> ("App.Kind"=w343:T12)  [unwired: 2 in, 2 out]
      n271 = case shown="\"Development System\"" w343 {
        tunnel: w342 -> [w348 _]
        frame "invalid app kind", Default {
          n272 = invoke on="Invoke Node" class="VI" method="FP.Close"(reference=w348) -> ()  [unwired: 2 in, 3 out]
        }
        frame "Development System" {
        }
      }
    }
  }
